vi "TCP IP Parse EnergyChannelId.vi"(11 "JSON in":string) -> (2 "Energy Channel ID":string, 3 "JSON out":string)   [LabVIEW 2015]
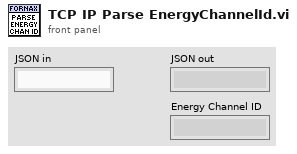
[diagram p1: front panel]
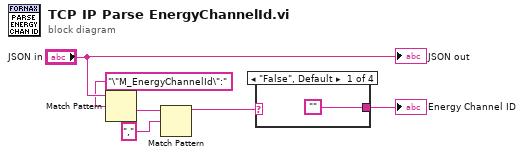
[diagram p0: block diagram]
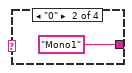
[diagram p2: hidden frame]
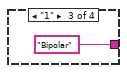
[diagram p3: hidden frame]
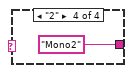
[diagram p4: hidden frame]
diagram:
  n1 = Match Pattern(string="JSON in", regular expression="\"M_EnergyChannelId\":") -> (after substring=w3:string)  [unwired: 1 in, 3 out]
  n2 = Match Pattern(string=w3, regular expression=",") -> (before substring=w1:string)  [unwired: 1 in, 3 out]
  n3 = case shown="\"False\", Default" w1 {
    tunnel: ["" "Mono1" ("regular expression") "Bipolar" ("regular expression") "Mono2" ("regular expression")] -> w6
    frame "False", Default {
    }
    frame "0" {
    }
    frame "1" {
    }
    frame "2" {
    }
  }
  "Energy Channel ID" <- w6
  "JSON out" <- "JSON in"
